vi "setEnableSpeedCtrl_ShootDualTalonSRX.vi"(9 "Enable Speed Control":bool) -> ()   [LabVIEW 2019, in "ShootDualTalonSRX_Motor_Pair.lvlib"]
uses:
  ShootDualTalonSRX_Motor_Pair.lvlib
  globals_ShootDualTalonSRX.vi
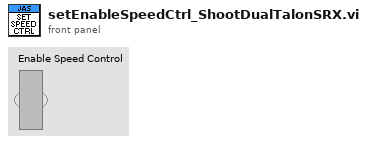
[diagram p1: front panel]
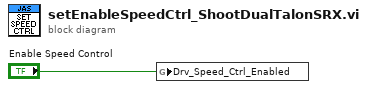
[diagram p0: block diagram]
diagram:
  n1 = global write "globals_ShootDualTalonSRX.vi" "Drv_Speed_Ctrl_Enabled"("Enable Speed Control") -> ()
